vi "Grouped Channel History (unix ns).vi"(4 "End":dbl, 6 "Start":dbl, 10 "Grouped Channels":T3, 11 "Historian Module in":refnum<class "Historian Module.lvclass">) -> (2 "History Data":T1, 3 "Historian Module out":refnum<class "Historian Module.lvclass">)   [LabVIEW 2020, in "VolatusHistorian.lvlib" / "Historian Module.lvclass"]
uses:
  Historian Module.lvclass
  History Data (unix ns).ctl
  Channel History (unix ns).ctl
  Historian Module.lvclass/Historian Module.ctl
  Time Filter Data (unix ns).vi
  lv-vecto/Vecto/Double Timestamp to Unix ns (Array).vi
  lv-vecto/Vecto/Double to Relative ns (Array).vi
  Group Buffer DBL/Data.vi
  VolatusHistorian.lvlib
  Grouped Channels.ctl
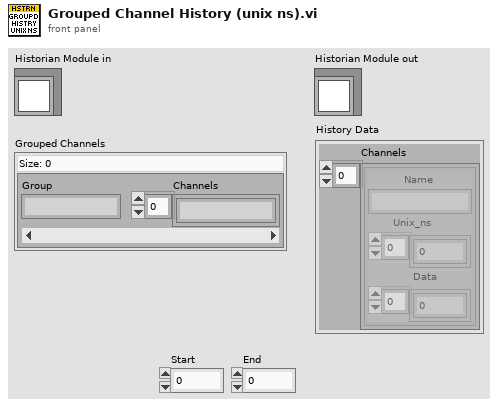
[diagram p1: front panel]
types:
  T1 = typedef "VolatusHistorian.lvlib/History Data (unix ns).ctl" = cluster{"Channels":T2[]}
  T2 = typedef "VolatusHistorian.lvlib/Channel History (unix ns).ctl" = cluster{"Name":string, "Unix_ns":i64[], "Data":dbl[]}
  T3 = typedef "VolatusHistorian.lvlib/Historian Module.lvclass/Grouped Channels.ctl" = map{string, string[]}
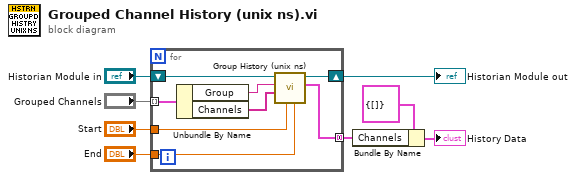
[diagram p0: block diagram]
diagram:
  n1 = for {
    tunnel: "Grouped Channels" -> [w15] mode=indexing
    tunnel: "Start" -> [w11]
    tunnel: "End" -> [w10]
    shift-right: [w14] -> w4
    shift-left: "Historian Module in" -> [w16]
    tunnel: [w9] -> w1 mode=concatenating
    n2 = Unbundle By Name(w15) -> ("Group"=w13:string, "Channels"=w12:string[])
    n3 = call "Group History (unix ns).vi"("End"=w10, "Start"=w11, "Channels"=w12, "Group"=w13, "Historian Module in"=w16) -> ("Data"=w9:T2[], "Historian Module out"=w14:refnum<class "Historian Module.lvclass">)  [unwired: 5 in]
  }
  "Historian Module out" <- w4
  n4 = Bundle By Name(cluster=T1 {"Channels"=[]} ("History Data"), "Channels"=w1) -> (→"History Data":T1)
